vi "0-Rotate Boat Overlays.vi"(3 "Overlay References In":T1, 4 "Sail Position":T3=0.5, 5 "Heading":T4 format="%05.1f") -> (1 "Rotated Boat Icon Bitmap Out":u32[][](array[colorbox]), 2 "Boat Icon Out":T2(plugin-control))   [LabVIEW 2011]
doc: "Rotates icon images of the boat and sails and overlays them on each other to create a representation of the current state of the robot. Also converts the output image to a bitmap for easy overlay on the mission map.\n\nby Jason Curtis"
uses:
  2-Think/2 Typedefs/heading.ctl
  2-Think/2 Typedefs/sail setpt.ctl
  0 Typedefs/Overlay References.ctl
  <vilib>/vision/Image Controls.llb/IMAQ Image.ctl
  <vilib>/vision/NI_Vision_Development_Module.lvlib
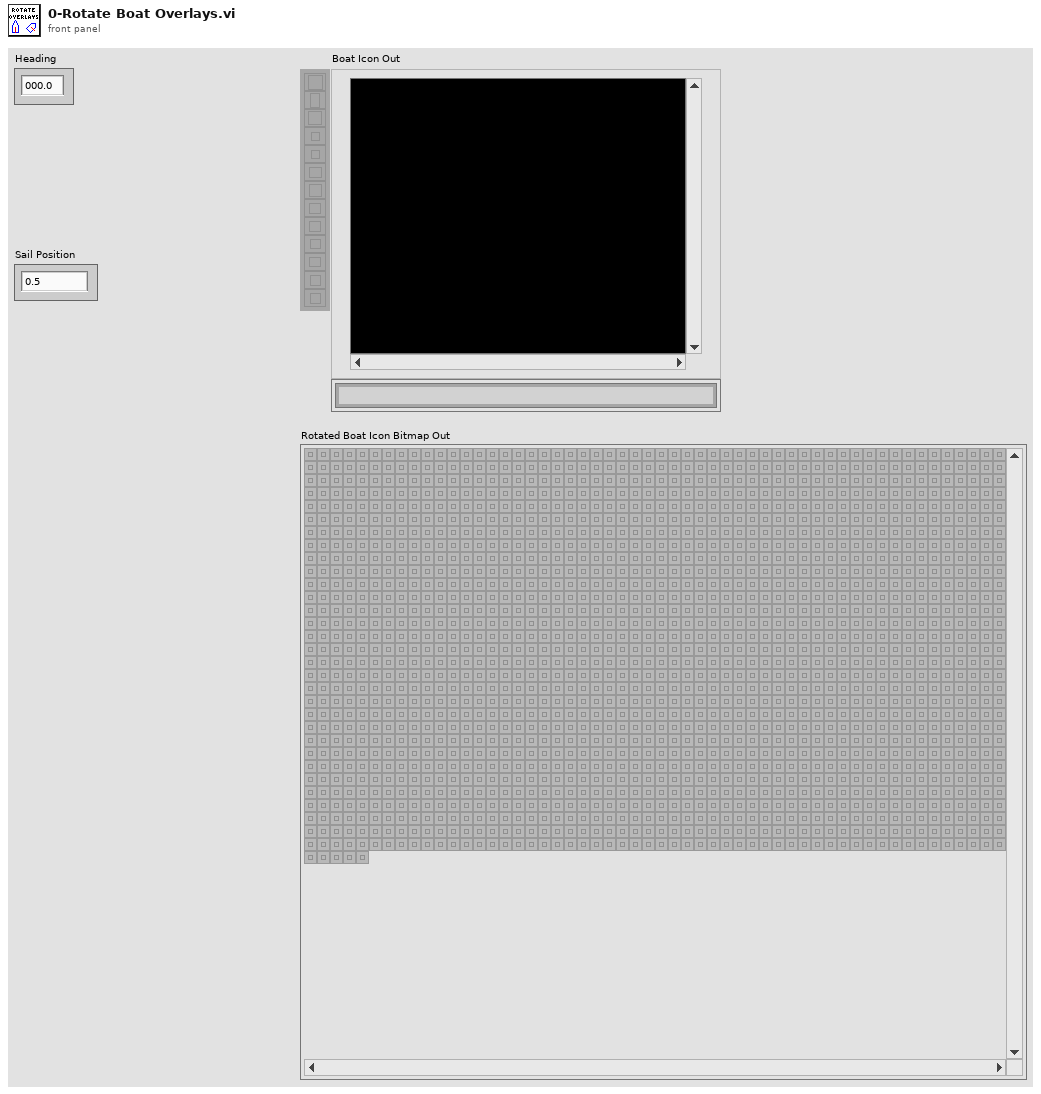
[diagram p1: front panel]
types:
  T1 = typedef "Overlay References.ctl" = cluster{"Boat Icon, Unroatated":T2, "Boat Icon, Rotated":T2, "Sail Icon, Unrotated":T2, "Sail Icon, Rotated":T2}
  T2 = typedef "IMAQ Image.ctl" = refnum<image>
  T3 = typedef "sail setpt.ctl" = dbl
  T4 = typedef "heading.ctl" = dbl
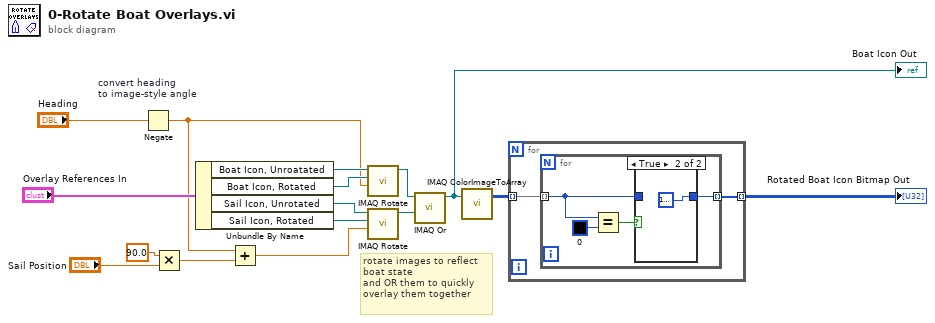
[diagram p0: block diagram]
diagram:
  # "rotate images to reflect\nboat state\nand OR them to quickly \noverlay them together"
  n1 = Negate "convert heading\nto image-style angle"(x="Heading") -> (-x=w3:T4)
  n2 = Multiply(x=T4 90.0 ("Heading 2"), y="Sail Position") -> (x*y=w4:T4)
  n3 = Unbundle By Name("Overlay References In") -> ("Boat Icon, Unroatated"=w16:T2, "Boat Icon, Rotated"=w15:T2, "Sail Icon, Unrotated"=w13:T2, "Sail Icon, Rotated"=w14:T2)
  n4 = Add(x=w3, y=w4) -> (x+y=w6:T4)
  n5 = call "IMAQ Rotate"("Angle (degrees)"=w3, "Image Dst"=w15, "Image Src"=w16) -> ("Image Dst Out"=w9:T2)  [unwired: 7 in, 1 out]
  n6 = call "IMAQ Rotate"("Angle (degrees)"=w6, "Image Dst"=w14, "Image Src"=w13) -> ("Image Dst Out"=w10:T2)  [unwired: 7 in, 1 out]
  n7 = call "IMAQ Or"("Image Src B"=w10, "Image Src A"=w9) -> ("Image Dst Out"=w11:T2)  [unwired: 8 in, 1 out]
  "Boat Icon Out" <- w11
  n8 = call "IMAQ ColorImageToArray"("Image"=w11) -> ("Image Pixels (U32)"=w7:u32[][])  [unwired: 2 in, 3 out]
  n9 = for {
    tunnel: w7 -> [w18] mode=indexing
    tunnel: [w17] -> w8 mode=indexing
    n10 = for {
      tunnel: w18 -> [w20] mode=indexing
      tunnel: [w21] -> w17 mode=indexing
      n11 = Equal?(x=w20, y=u32 0) -> (x = y?=w22:bool)
      n12 = case shown="True" w22 {
        tunnel: [w23 u32 16777216] -> w21
        tunnel: w20 -> [w23 _]
        frame False {
        }
        frame True {
        }
      }
    }
  }
  "Rotated Boat Icon Bitmap Out" <- w8
